vi "S4GUI_003.vi"(7 "Tab ObsEng":enum32{"Obs", "CCD modes", "Guider", "Eng"}(tab)) -> ()   [LabVIEW 2018] (continued)
            n4414 = call-dynamic "Read Channel.vi"("error in (no error)"=w10358, "Acquisition in"=w10359) -> ("error out"=w10342:errorcluster, "Channel.lvclass"=w10346:refnum<class "Channel.lvclass">, "Acquisition out"=w10352:refnum<class "Acquisition.lvclass">)  [unwired: 7 in]
            n4415 = call-dynamic "Read Interface.vi"("error in (no error)"=w10342, "Channel in"=w10346) -> ("error out"=w10337:errorcluster, "Interface.lvclass"=w10338:refnum<class "Interface.lvclass">, "Channel out"=w10345:refnum<class "Channel.lvclass">)  [unwired: 7 in]
            n4416 = call-dynamic "Write Cooler ON_OFF.vi"("error in (no error)"=w10337, "Cooler ON/OFF"=w10329, "Interface in"=w10338) -> ("error out"=w10341:errorcluster, "Interface out"=w10343:refnum<class "Interface.lvclass">)  [unwired: 7 in]
            n4417 = call-dynamic "Write Interface.vi"("error in (no error)"=w10341, "Interface.lvclass"=w10343, "Channel in"=w10345) -> ("error out"=w10340:errorcluster, "Channel out"=w10344:refnum<class "Channel.lvclass">)  [unwired: 7 in]
            n4418 = call-dynamic "Read State Machine.vi"("error in (no error)"=w10340, "Device in"=w10344) -> ("error out"=w10356:errorcluster, "State Machine.lvclass"=w10357:refnum<class "State Machine.lvclass">, "Device out"=w10353:refnum<class "Channel.lvclass">)  [unwired: 7 in]
            n4419 = call "Next State.vi"("error in (no error)"=w10356, "New_State"=u32 30, "State Machine in"=w10357) -> ("error out"=w10351:errorcluster, "State Machine out"=w10354:refnum<class "State Machine.lvclass">)  [unwired: 7 in]
            n4420 = call-dynamic "Write State Machine.vi"("error in (no error)"=w10351, "State Machine.lvclass"=w10354, "Device in"=w10353) -> ("error out"=w10347:errorcluster, "Device out"=w10339:refnum<class "Channel.lvclass">)  [unwired: 7 in]
            n4421 = call-dynamic "Write Channel.vi"("error in (no error)"=w10347, "Channel.lvclass"=w10339, "Acquisition in"=w10352) -> ("error out"=w10348:errorcluster, "Acquisition out"=w10350:refnum<class "Acquisition.lvclass">)  [unwired: 7 in]
            n4422 = call-dynamic "Write AcquisitionD.vi"("error in (no error)"=w10348, "Acquisition.lvclass"=w10350, "S4ACS_GUI in"=w10349) -> ("error out"=w10361:errorcluster, "S4ACS_GUI out"=w10360:refnum<class "S4GUI.lvclass">)  [unwired: 7 in]
          }
        }
      }
      event "Set Temp 1": Value Change {
        n4423 = event-data() -> ("NewVal"=w10362:bool)  [unwired: 1 in]
        n4424 = case shown="True" w10362 {
          tunnel: w10366 -> [w10368 w10385]
          tunnel: w10365 -> [w10367 w10384]
          tunnel: [w10367 w10374] -> w10364
          tunnel: [w10368 w10375] -> w10363
          frame False {
          }
          frame True {
            # "Carrega a maior temperatura\nentre target atual e o target do controle."
            # "Carrega o valor da temperatura target de acordo com a conf CCD"
            n4425 = call-dynamic "Read AcquisitionA.vi"("error in (no error)"=w10384, "S4ACS_GUI in"=w10385) -> ("error out"=w10387:errorcluster, "Acquisition.lvclass"=w10386:refnum<class "Acquisition.lvclass">, "S4ACS_GUI out"=w10371:refnum<class "S4GUI.lvclass">)  [unwired: 7 in]
            n4426 = call-dynamic "Read Channel.vi"("error in (no error)"=w10387, "Acquisition in"=w10386) -> ("error out"=w10398:errorcluster, "Channel.lvclass"=w10397:refnum<class "Channel.lvclass">, "Acquisition out"=w10370:refnum<class "Acquisition.lvclass">)  [unwired: 7 in]
            n4427 = call-dynamic "ValidateConfig.vi"("error in (no error)"=w10398, "Channel in"=w10397) -> ("error out"=w10404:errorcluster, "Channel out"=w10403:refnum<class "Channel.lvclass">)  [unwired: 7 in, 1 out]
            n4428 = call-dynamic "Read Interface.vi"("error in (no error)"=w10404, "Channel in"=w10403) -> ("error out"=w10400:errorcluster, "Interface.lvclass"=w10399:refnum<class "Interface.lvclass">, "Channel out"=w10393:refnum<class "Channel.lvclass">)  [unwired: 7 in]
            n4429 = call-dynamic "Read Temperature.vi"("error in (no error)"=w10400, "Interface in"=w10399) -> ("error out"=w10401:errorcluster, "Temperature"=w10405:i8, "Interface out"=w10402:refnum<class "Interface.lvclass">)  [unwired: 7 in]
            n4430 = Greater?(x=w10405, y="Target Temp 1") -> (0:w10373:bool)
            n4431 = Select(t=w10405, s=w10373, f="Target Temp 1") -> (s? t:f=w10378:i8)
            n4432 = call-dynamic "Write Temperature.vi"("error in (no error)"=w10401, "Temperature"=w10378, "Interface in"=w10402) -> ("error out"=w10395:errorcluster, "Interface out"=w10392:refnum<class "Interface.lvclass">)  [unwired: 7 in]
            n4433 = call-dynamic "Write Interface.vi"("error in (no error)"=w10395, "Interface.lvclass"=w10392, "Channel in"=w10393) -> ("error out"=w10396:errorcluster, "Channel out"=w10394:refnum<class "Channel.lvclass">)  [unwired: 7 in]
            n4434 = case shown="True" w10373 {
              tunnel: w10396 -> [w10430 w10433]
              tunnel: w10394 -> [w10429 w10440]
              tunnel: [w10428 w10440] -> w10391
              tunnel: [w10427 w10439] -> w10390
              tunnel: w10371 -> [w10407 w10435]
              tunnel: [w10407 w10438] -> w10372
              tunnel: w10370 -> [w10406 w10437]
              tunnel: [w10406 w10436] -> w10369
              frame False {
                # "input ok"
                n4435 = call-dynamic "Read State Machine.vi"("error in (no error)"=w10430, "Device in"=w10429) -> ("error out"=w10409:errorcluster, "State Machine.lvclass"=w10416:refnum<class "State Machine.lvclass">, "Device out"=w10425:refnum<class "Channel.lvclass">)  [unwired: 7 in]
                n4436 = call-dynamic "Read ref StatesQueue.vi"("error in (no error)"=w10409, "State Machine in"=w10416) -> ("error out"=w10419:errorcluster, "ref StatesQueue"=w10413:refnum<queue>, "State Machine out"=w10415:refnum<class "State Machine.lvclass">)  [unwired: 7 in]
                n4437 = Flush Queue(queue=w10413, error in (no error)=w10419) -> (queue out=w10412:refnum<queue>, error out=w10421:errorcluster)  [unwired: 1 out]
                n4438 = Enqueue Element(queue=w10412, element=u32 35 ("State"), error in (no error)=w10421) -> (queue out=w10411:refnum<queue>, error out=w10422:errorcluster)  [unwired: 1 in, 1 out]
                n4439 = Enqueue Element(queue=w10411, element=u32 37 ("State"), error in (no error)=w10422) -> (queue out=w10410:refnum<queue>, error out=w10420:errorcluster)  [unwired: 1 in, 1 out]
                n4440 = call-dynamic "Write ref StatesQueue.vi"("error in (no error)"=w10420, "ref StatesQueue"=w10410, "State Machine in"=w10415) -> ("error out"=w10408:errorcluster, "State Machine out"=w10414:refnum<class "State Machine.lvclass">)  [unwired: 7 in]
                n4441 = call "Next State.vi"("error in (no error)"=w10408, "New_State"=u32 0, "State Machine in"=w10414) -> ("error out"=w10426:errorcluster, "State Machine out"=w10424:refnum<class "State Machine.lvclass">)  [unwired: 7 in]
                n4442 = call-dynamic "Write State Machine.vi"("error in (no error)"=w10426, "State Machine.lvclass"=w10424, "Device in"=w10425) -> ("error out"=w10427:errorcluster, "Device out"=w10428:refnum<class "Channel.lvclass">)  [unwired: 7 in]
              }
              frame True {
                # "input error"
                n4443 = call-dynamic "Read SET temp error mode.vi"("error in (no error)"=w10433, "S4GUI in"=w10435) -> ("error out"=w10432:errorcluster, "SET temp error mode"=w10431:bool, "S4GUI out"=w10434:refnum<class "S4GUI.lvclass">)  [unwired: 7 in]
                n4444 = case shown="False" w10431 {
                  tunnel: [w10449 w10464] -> w10439
                  tunnel: [w10448 w10463] -> w10438
                  tunnel: w10434 -> [w10447 w10463]
                  tunnel: w10432 -> [w10444 w10465]
                  tunnel: w10437 -> [w10442 w10462]
                  tunnel: [w10441 w10462] -> w10436
                  frame False {
                    # "last error msg"
                    n4445 = call-dynamic "Read sync.vi"("error in (no error)"=w10444, "S4ACS_GUI in"=w10447) -> ("error out"=w10443:errorcluster, "sync"=w10445:bool, "S4ACS_GUI out"=w10446:refnum<class "S4GUI.lvclass">)  [unwired: 7 in]
                    n4446 = case shown="False" w10445 {
                      tunnel: w10443 -> [w10452 w10461]
                      tunnel: [w10451 w10460] -> w10449
                      tunnel: [w10455 w10459] -> w10448
                      tunnel: w10446 -> [w10455 w10457]
                      tunnel: w10442 -> [w10453 w10456]
                      tunnel: [w10450 w10456] -> w10441
                      frame False {
                        n4447 = call-dynamic "Write Acq_state.vi"("error in (no error)"=w10452, "Acq_state"=u32 240, "Acquisition in"=w10453) -> ("error out"=w10451:errorcluster, "Acquisition out"=w10450:refnum<class "Acquisition.lvclass">)  [unwired: 7 in]
                      }
                      frame True {
                        n4448 = call-dynamic "Write Obs_state.vi"("error in (no error)"=w10461, "Obs_state"=u32 240, "S4ACS_GUI in"=w10457) -> ("error out"=w10460:errorcluster, "S4ACS_GUI out"=w10459:refnum<class "S4GUI.lvclass">)  [unwired: 7 in]
                      }
                    }
                  }
                  frame True {
                    # "popup msg"
                    n4449 = disable-structure shown="Enabled" {
                      disable-tunnel: w10465 -> [w10467 w10474]
                      disable-tunnel: [w10466 w10474] -> w10464
                      frame Enabled {
                        w10469 = FALSE ("Wait Until Done")
                        n4450 = call <vilib>:"Application Directory.vi"() -> ("Application Directory"=w10473:path)
                        n4451 = Build Path(base path=w10473, name or relative path="MsgSetTemp.vi") -> (appended path=w10470:path)
                        n4452 = Open VI Reference(vi path=w10470, error in (no error)=w10467) -> (vi reference=w10471:refnum<vi>, error out=w10472:errorcluster)  [unwired: 4 in]
                        n4453 = invoke class="VI" method="Run VI"(reference=w10471, error in=w10472, "Wait until done"=w10469, "Auto Dispose Ref"=w10469) -> (error out=w10466:errorcluster)  [unwired: 1 in, 4 out]
                      }
                      frame Disabled {
                        n4454 = One Button Dialog(message="ERROR: Invalid input value. It must be \nequal or greater than the minimum for \nthe current CCD setup.", button name ("OK")="OK" ("T button name (\"OK\")")) -> ()  [unwired: 1 out]
                      }
                    }
                  }
                }
              }
            }
            n4455 = Number To Decimal String(number="Target Temp 1") -> (decimal integer string=w10377:string)  [unwired: 1 in]
            n4456 = call-dynamic "Write Channel.vi"("error in (no error)"=w10390, "Channel.lvclass"=w10391, "Acquisition in"=w10369) -> ("error out"=w10389:errorcluster, "Acquisition out"=w10388:refnum<class "Acquisition.lvclass">)  [unwired: 7 in]
            n4457 = Concatenate Strings("SET TEMP [" ("User Event"), w10377, "] CLICKED - CH1" ("User Event")) -> (w10383:string)
            n4458 = call-dynamic "Write AcquisitionA.vi"("error in (no error)"=w10389, "Acquisition.lvclass"=w10388, "S4ACS_GUI in"=w10372) -> ("error out"=w10379:errorcluster, "S4ACS_GUI out"=w10380:refnum<class "S4GUI.lvclass">)  [unwired: 7 in]
            n4459 = call-dynamic "Write User Event.vi"("error in (no error)"=w10379, "User Event"=w10383, "S4GUI in"=w10380) -> ("error out"=w10374:errorcluster, "S4GUI out"=w10375:refnum<class "S4GUI.lvclass">)  [unwired: 7 in]
          }
        }
      }
      event "Set Temp 2": Value Change {
        n4460 = event-data() -> ("NewVal"=w10477:bool)  [unwired: 1 in]
        n4461 = case shown="True" w10477 {
          tunnel: w10481 -> [w10483 w10503]
          tunnel: w10480 -> [w10482 w10502]
          tunnel: [w10482 w10495] -> w10479
          tunnel: [w10483 w10497] -> w10478
          frame False {
          }
          frame True {
            # "Carrega a maior temperatura\nentre target atual e o target do controle."
            # "Carrega o valor da temperatura target de acordo com a conf CCD"
            n4462 = call "Read AcquisitionB.vi"("error in (no error)"=w10502, "S4ACS_GUI in"=w10503) -> ("error out"=w10519:errorcluster, "Acquisition.lvclass"=w10520:refnum<class "Acquisition.lvclass">, "S4ACS_GUI out"=w10490:refnum<class "S4GUI.lvclass">)  [unwired: 7 in]
            n4463 = call-dynamic "Read Channel.vi"("error in (no error)"=w10519, "Acquisition in"=w10520) -> ("error out"=w10512:errorcluster, "Channel.lvclass"=w10513:refnum<class "Channel.lvclass">, "Acquisition out"=w10491:refnum<class "Acquisition.lvclass">)  [unwired: 7 in]
            n4464 = call-dynamic "ValidateConfig.vi"("error in (no error)"=w10512, "Channel in"=w10513) -> ("error out"=w10506:errorcluster, "Channel out"=w10507:refnum<class "Channel.lvclass">)  [unwired: 7 in, 1 out]
            n4465 = call-dynamic "Read Interface.vi"("error in (no error)"=w10506, "Channel in"=w10507) -> ("error out"=w10510:errorcluster, "Interface.lvclass"=w10511:refnum<class "Interface.lvclass">, "Channel out"=w10515:refnum<class "Channel.lvclass">)  [unwired: 7 in]
            n4466 = call-dynamic "Read Temperature.vi"("error in (no error)"=w10510, "Interface in"=w10511) -> ("error out"=w10509:errorcluster, "Temperature"=w10505:i8, "Interface out"=w10508:refnum<class "Interface.lvclass">)  [unwired: 7 in]
            n4467 = Greater?(x=w10505, y="Target Temp 2") -> (0:w10488:bool)
            n4468 = Select(t=w10505, s=w10488, f="Target Temp 2") -> (s? t:f=w10504:i32)
            n4469 = call-dynamic "Write Temperature.vi"("error in (no error)"=w10509, "Temperature"=w10504, "Interface in"=w10508) -> ("error out"=w10514:errorcluster, "Interface out"=w10516:refnum<class "Interface.lvclass">)  [unwired: 7 in]
            n4470 = call-dynamic "Write Interface.vi"("error in (no error)"=w10514, "Interface.lvclass"=w10516, "Channel in"=w10515) -> ("error out"=w10489:errorcluster, "Channel out"=w10492:refnum<class "Channel.lvclass">)  [unwired: 7 in]
            n4471 = case shown="True" w10488 {
              tunnel: w10489 -> [w10545 w10550]
              tunnel: w10492 -> [w10544 w10552]
              tunnel: [w10543 w10552] -> w10485
              tunnel: [w10542 w10555] -> w10484
              tunnel: w10490 -> [w10522 w10551]
              tunnel: [w10522 w10554] -> w10487
              tunnel: w10491 -> [w10521 w10546]
              tunnel: [w10521 w10553] -> w10486
              frame False {
                # "input ok"
                n4472 = call-dynamic "Read State Machine.vi"("error in (no error)"=w10545, "Device in"=w10544) -> ("error out"=w10524:errorcluster, "State Machine.lvclass"=w10531:refnum<class "State Machine.lvclass">, "Device out"=w10540:refnum<class "Channel.lvclass">)  [unwired: 7 in]
                n4473 = call-dynamic "Read ref StatesQueue.vi"("error in (no error)"=w10524, "State Machine in"=w10531) -> ("error out"=w10534:errorcluster, "ref StatesQueue"=w10528:refnum<queue>, "State Machine out"=w10530:refnum<class "State Machine.lvclass">)  [unwired: 7 in]
                n4474 = Flush Queue(queue=w10528, error in (no error)=w10534) -> (queue out=w10527:refnum<queue>, error out=w10536:errorcluster)  [unwired: 1 out]
                n4475 = Enqueue Element(queue=w10527, element=u32 35 ("State"), error in (no error)=w10536) -> (queue out=w10526:refnum<queue>, error out=w10537:errorcluster)  [unwired: 1 in, 1 out]
                n4476 = Enqueue Element(queue=w10526, element=u32 37 ("State"), error in (no error)=w10537) -> (queue out=w10525:refnum<queue>, error out=w10535:errorcluster)  [unwired: 1 in, 1 out]
                n4477 = call-dynamic "Write ref StatesQueue.vi"("error in (no error)"=w10535, "ref StatesQueue"=w10525, "State Machine in"=w10530) -> ("error out"=w10523:errorcluster, "State Machine out"=w10529:refnum<class "State Machine.lvclass">)  [unwired: 7 in]
                n4478 = call "Next State.vi"("error in (no error)"=w10523, "New_State"=u32 0, "State Machine in"=w10529) -> ("error out"=w10541:errorcluster, "State Machine out"=w10539:refnum<class "State Machine.lvclass">)  [unwired: 7 in]
                n4479 = call-dynamic "Write State Machine.vi"("error in (no error)"=w10541, "State Machine.lvclass"=w10539, "Device in"=w10540) -> ("error out"=w10542:errorcluster, "Device out"=w10543:refnum<class "Channel.lvclass">)  [unwired: 7 in]
              }
              frame True {
                # "input error"
                n4480 = call-dynamic "Read SET temp error mode.vi"("error in (no error)"=w10550, "S4GUI in"=w10551) -> ("error out"=w10547:errorcluster, "SET temp error mode"=w10549:bool, "S4GUI out"=w10548:refnum<class "S4GUI.lvclass">)  [unwired: 7 in]
                n4481 = case shown="False" w10549 {
                  tunnel: [w10564 w10577] -> w10555
                  tunnel: [w10563 w10586] -> w10554
                  tunnel: [w10559 w10585] -> w10553
                  tunnel: w10546 -> [w10558 w10585]
                  tunnel: w10548 -> [w10557 w10586]
                  tunnel: w10547 -> [w10556 w10578]
                  frame False {
                    # "last error msg"
                    n4482 = call-dynamic "Read sync.vi"("error in (no error)"=w10556, "S4ACS_GUI in"=w10557) -> ("error out"=w10560:errorcluster, "sync"=w10561:bool, "S4ACS_GUI out"=w10562:refnum<class "S4GUI.lvclass">)  [unwired: 7 in]
                    n4483 = case shown="True" w10561 {
                      tunnel: w10560 -> [w10567 w10576]
                      tunnel: [w10566 w10575] -> w10564
                      tunnel: [w10570 w10574] -> w10563
                      tunnel: w10562 -> [w10570 w10572]
                      tunnel: w10558 -> [w10568 w10571]
                      tunnel: [w10565 w10571] -> w10559
                      frame False {
                        n4484 = call-dynamic "Write Acq_state.vi"("error in (no error)"=w10567, "Acq_state"=u32 240, "Acquisition in"=w10568) -> ("error out"=w10566:errorcluster, "Acquisition out"=w10565:refnum<class "Acquisition.lvclass">)  [unwired: 7 in]
                      }
                      frame True {
                        n4485 = call-dynamic "Write Obs_state.vi"("error in (no error)"=w10576, "Obs_state"=u32 240, "S4ACS_GUI in"=w10572) -> ("error out"=w10575:errorcluster, "S4ACS_GUI out"=w10574:refnum<class "S4GUI.lvclass">)  [unwired: 7 in]
                      }
                    }
                  }
                  frame True {
                    w10580 = FALSE ("Wait Until Done")
                    # "popup msg"
                    n4486 = call <vilib>:"Application Directory.vi"() -> ("Application Directory"=w10584:path)
                    n4487 = Build Path(base path=w10584, name or relative path="MsgSetTemp.vi") -> (appended path=w10581:path)
                    n4488 = Open VI Reference(vi path=w10581, error in (no error)=w10578) -> (vi reference=w10582:refnum<vi>, error out=w10583:errorcluster)  [unwired: 4 in]
                    n4489 = invoke class="VI" method="Run VI"(reference=w10582, error in=w10583, "Wait until done"=w10580, "Auto Dispose Ref"=w10580) -> (error out=w10577:errorcluster)  [unwired: 1 in, 4 out]
                  }
                }
              }
            }
            n4490 = Number To Decimal String(number="Target Temp 2") -> (decimal integer string=w10493:string)  [unwired: 1 in]
            n4491 = call-dynamic "Write Channel.vi"("error in (no error)"=w10484, "Channel.lvclass"=w10485, "Acquisition in"=w10486) -> ("error out"=w10517:errorcluster, "Acquisition out"=w10518:refnum<class "Acquisition.lvclass">)  [unwired: 7 in]
            n4492 = Concatenate Strings("SET TEMP [" ("User Event"), w10493, "] CLICKED - CH2" ("User Event")) -> (w10501:string)
            n4493 = call "Write AcquisitionB.vi"("error in (no error)"=w10517, "Acquisition.lvclass"=w10518, "S4ACS_GUI in"=w10487) -> ("error out"=w10496:errorcluster, "S4ACS_GUI out"=w10498:refnum<class "S4GUI.lvclass">)  [unwired: 7 in]
            n4494 = call-dynamic "Write User Event.vi"("error in (no error)"=w10496, "User Event"=w10501, "S4GUI in"=w10498) -> ("error out"=w10495:errorcluster, "S4GUI out"=w10497:refnum<class "S4GUI.lvclass">)  [unwired: 7 in]
          }
        }
      }
      event "Set Temp 3": Value Change {
        n4495 = event-data() -> ("NewVal"=w10587:bool)  [unwired: 1 in]
        n4496 = case shown="True" w10587 {
          tunnel: w10591 -> [w10593 w10613]
          tunnel: w10590 -> [w10592 w10612]
          tunnel: [w10592 w10604] -> w10589
          tunnel: [w10593 w10606] -> w10588
          frame False {
          }
          frame True {
            # "Carrega a maior temperatura\nentre target atual e o target do controle."
            # "Carrega o valor da temperatura target de acordo com a conf CCD"
            n4497 = call-dynamic "Read AcquisitionC.vi"("error in (no error)"=w10612, "S4ACS_GUI in"=w10613) -> ("error out"=w10615:errorcluster, "Acquisition.lvclass"=w10614:refnum<class "Acquisition.lvclass">, "S4ACS_GUI out"=w10595:refnum<class "S4GUI.lvclass">)  [unwired: 7 in]
            n4498 = call-dynamic "Read Channel.vi"("error in (no error)"=w10615, "Acquisition in"=w10614) -> ("error out"=w10622:errorcluster, "Channel.lvclass"=w10621:refnum<class "Channel.lvclass">, "Acquisition out"=w10596:refnum<class "Acquisition.lvclass">)  [unwired: 7 in]
            n4499 = call-dynamic "ValidateConfig.vi"("error in (no error)"=w10622, "Channel in"=w10621) -> ("error out"=w10628:errorcluster, "Channel out"=w10627:refnum<class "Channel.lvclass">)  [unwired: 7 in, 1 out]
            n4500 = call-dynamic "Read Interface.vi"("error in (no error)"=w10628, "Channel in"=w10627) -> ("error out"=w10624:errorcluster, "Interface.lvclass"=w10623:refnum<class "Interface.lvclass">, "Channel out"=w10619:refnum<class "Channel.lvclass">)  [unwired: 7 in]
            n4501 = call-dynamic "Read Temperature.vi"("error in (no error)"=w10624, "Interface in"=w10623) -> ("error out"=w10625:errorcluster, "Temperature"=w10629:i8, "Interface out"=w10626:refnum<class "Interface.lvclass">)  [unwired: 7 in]
            n4502 = Greater?(x=w10629, y="Target Temp 3") -> (0:w10594:bool)
            n4503 = Select(t=w10629, s=w10594, f="Target Temp 3") -> (s? t:f=w10630:i32)
            n4504 = call-dynamic "Write Temperature.vi"("error in (no error)"=w10625, "Temperature"=w10630, "Interface in"=w10626) -> ("error out"=w10620:errorcluster, "Interface out"=w10618:refnum<class "Interface.lvclass">)  [unwired: 7 in]
            n4505 = call-dynamic "Write Interface.vi"("error in (no error)"=w10620, "Interface.lvclass"=w10618, "Channel in"=w10619) -> ("error out"=w10597:errorcluster, "Channel out"=w10602:refnum<class "Channel.lvclass">)  [unwired: 7 in]
            n4506 = case shown="True" w10594 {
              tunnel: w10597 -> [w10655 w10656]
              tunnel: w10602 -> [w10654 w10662]
              tunnel: [w10653 w10662] -> w10601
              tunnel: [w10652 w10665] -> w10598
              tunnel: w10595 -> [w10632 w10661]
              tunnel: [w10632 w10664] -> w10599
              tunnel: w10596 -> [w10631 w10659]
              tunnel: [w10631 w10663] -> w10600
              frame False {
                # "input ok"
                n4507 = call-dynamic "Read State Machine.vi"("error in (no error)"=w10655, "Device in"=w10654) -> ("error out"=w10634:errorcluster, "State Machine.lvclass"=w10641:refnum<class "State Machine.lvclass">, "Device out"=w10650:refnum<class "Channel.lvclass">)  [unwired: 7 in]
                n4508 = call-dynamic "Read ref StatesQueue.vi"("error in (no error)"=w10634, "State Machine in"=w10641) -> ("error out"=w10644:errorcluster, "ref StatesQueue"=w10638:refnum<queue>, "State Machine out"=w10640:refnum<class "State Machine.lvclass">)  [unwired: 7 in]
                n4509 = Flush Queue(queue=w10638, error in (no error)=w10644) -> (queue out=w10637:refnum<queue>, error out=w10646:errorcluster)  [unwired: 1 out]
                n4510 = Enqueue Element(queue=w10637, element=u32 35 ("State"), error in (no error)=w10646) -> (queue out=w10636:refnum<queue>, error out=w10647:errorcluster)  [unwired: 1 in, 1 out]
                n4511 = Enqueue Element(queue=w10636, element=u32 37 ("State"), error in (no error)=w10647) -> (queue out=w10635:refnum<queue>, error out=w10645:errorcluster)  [unwired: 1 in, 1 out]
                n4512 = call-dynamic "Write ref StatesQueue.vi"("error in (no error)"=w10645, "ref StatesQueue"=w10635, "State Machine in"=w10640) -> ("error out"=w10633:errorcluster, "State Machine out"=w10639:refnum<class "State Machine.lvclass">)  [unwired: 7 in]
                n4513 = call "Next State.vi"("error in (no error)"=w10633, "New_State"=u32 0, "State Machine in"=w10639) -> ("error out"=w10651:errorcluster, "State Machine out"=w10649:refnum<class "State Machine.lvclass">)  [unwired: 7 in]
                n4514 = call-dynamic "Write State Machine.vi"("error in (no error)"=w10651, "State Machine.lvclass"=w10649, "Device in"=w10650) -> ("error out"=w10652:errorcluster, "Device out"=w10653:refnum<class "Channel.lvclass">)  [unwired: 7 in]
              }
              frame True {
                # "input error"
                n4515 = call-dynamic "Read SET temp error mode.vi"("error in (no error)"=w10656, "S4GUI in"=w10661) -> ("error out"=w10657:errorcluster, "SET temp error mode"=w10658:bool, "S4GUI out"=w10660:refnum<class "S4GUI.lvclass">)  [unwired: 7 in]
                n4516 = case shown="False" w10658 {
                  tunnel: [w10674 w10687] -> w10665
                  tunnel: [w10673 w10696] -> w10664
                  tunnel: w10660 -> [w10672 w10696]
                  tunnel: w10657 -> [w10669 w10688]
                  tunnel: w10659 -> [w10667 w10695]
                  tunnel: [w10666 w10695] -> w10663
                  frame False {
                    # "last error msg"
                    n4517 = call-dynamic "Read sync.vi"("error in (no error)"=w10669, "S4ACS_GUI in"=w10672) -> ("error out"=w10668:errorcluster, "sync"=w10670:bool, "S4ACS_GUI out"=w10671:refnum<class "S4GUI.lvclass">)  [unwired: 7 in]
                    n4518 = case shown="True" w10670 {
                      tunnel: w10668 -> [w10677 w10686]
                      tunnel: [w10676 w10685] -> w10674
                      tunnel: [w10680 w10684] -> w10673
                      tunnel: w10671 -> [w10680 w10682]
                      tunnel: w10667 -> [w10678 w10681]
                      tunnel: [w10675 w10681] -> w10666
                      frame False {
                        n4519 = call-dynamic "Write Acq_state.vi"("error in (no error)"=w10677, "Acq_state"=u32 240, "Acquisition in"=w10678) -> ("error out"=w10676:errorcluster, "Acquisition out"=w10675:refnum<class "Acquisition.lvclass">)  [unwired: 7 in]
                      }
                      frame True {
                        n4520 = call-dynamic "Write Obs_state.vi"("error in (no error)"=w10686, "Obs_state"=u32 240, "S4ACS_GUI in"=w10682) -> ("error out"=w10685:errorcluster, "S4ACS_GUI out"=w10684:refnum<class "S4GUI.lvclass">)  [unwired: 7 in]
                      }
                    }
                  }
                  frame True {
                    w10690 = FALSE ("Wait Until Done")
                    # "popup msg"
                    n4521 = call <vilib>:"Application Directory.vi"() -> ("Application Directory"=w10691:path)
                    n4522 = Build Path(base path=w10691, name or relative path="MsgSetTemp.vi") -> (appended path=w10694:path)
                    n4523 = Open VI Reference(vi path=w10694, error in (no error)=w10688) -> (vi reference=w10693:refnum<vi>, error out=w10692:errorcluster)  [unwired: 4 in]
                    n4524 = invoke class="VI" method="Run VI"(reference=w10693, error in=w10692, "Wait until done"=w10690, "Auto Dispose Ref"=w10690) -> (error out=w10687:errorcluster)  [unwired: 1 in, 4 out]
                  }
                }
              }
            }
            n4525 = Number To Decimal String(number="Target Temp 3") -> (decimal integer string=w10608:string)  [unwired: 1 in]
            n4526 = call-dynamic "Write Channel.vi"("error in (no error)"=w10598, "Channel.lvclass"=w10601, "Acquisition in"=w10600) -> ("error out"=w10617:errorcluster, "Acquisition out"=w10616:refnum<class "Acquisition.lvclass">)  [unwired: 7 in]
            n4527 = call-dynamic "Write AcquisitionC.vi"("error in (no error)"=w10617, "Acquisition.lvclass"=w10616, "S4ACS_GUI in"=w10599) -> ("error out"=w10605:errorcluster, "S4ACS_GUI out"=w10607:refnum<class "S4GUI.lvclass">)  [unwired: 7 in]
            n4528 = Concatenate Strings("SET TEMP [" ("User Event"), w10608, "] CLICKED - CH3" ("User Event")) -> (w10611:string)
            n4529 = call-dynamic "Write User Event.vi"("error in (no error)"=w10605, "User Event"=w10611, "S4GUI in"=w10607) -> ("error out"=w10604:errorcluster, "S4GUI out"=w10606:refnum<class "S4GUI.lvclass">)  [unwired: 7 in]
          }
        }
      }
      event "Set Temp 4": Value Change {
        n4530 = event-data() -> ("NewVal"=w10697:bool)  [unwired: 1 in]
        n4531 = case shown="True" w10697 {
          tunnel: w10701 -> [w10703 w10736]
          tunnel: w10700 -> [w10702 w10735]
          tunnel: [w10702 w10713] -> w10699
          tunnel: [w10703 w10714] -> w10698
          frame False {
          }
          frame True {
            # "Carrega a maior temperatura\nentre target atual e o target do controle."
            # "Carrega o valor da temperatura target de acordo com a conf CCD"
            n4532 = call-dynamic "Read AcquisitionD.vi"("error in (no error)"=w10735, "S4ACS_GUI in"=w10736) -> ("error out"=w10739:errorcluster, "Acquisition.lvclass"=w10740:refnum<class "Acquisition.lvclass">, "S4ACS_GUI out"=w10709:refnum<class "S4GUI.lvclass">)  [unwired: 7 in]
            n4533 = call-dynamic "Read Channel.vi"("error in (no error)"=w10739, "Acquisition in"=w10740) -> ("error out"=w10730:errorcluster, "Channel.lvclass"=w10731:refnum<class "Channel.lvclass">, "Acquisition out"=w10710:refnum<class "Acquisition.lvclass">)  [unwired: 7 in]
            n4534 = call-dynamic "ValidateConfig.vi"("error in (no error)"=w10730, "Channel in"=w10731) -> ("error out"=w10724:errorcluster, "Channel out"=w10725:refnum<class "Channel.lvclass">)  [unwired: 7 in, 1 out]
            n4535 = call-dynamic "Read Interface.vi"("error in (no error)"=w10724, "Channel in"=w10725) -> ("error out"=w10728:errorcluster, "Interface.lvclass"=w10729:refnum<class "Interface.lvclass">, "Channel out"=w10733:refnum<class "Channel.lvclass">)  [unwired: 7 in]
            n4536 = call-dynamic "Read Temperature.vi"("error in (no error)"=w10728, "Interface in"=w10729) -> ("error out"=w10727:errorcluster, "Temperature"=w10723:i8, "Interface out"=w10726:refnum<class "Interface.lvclass">)  [unwired: 7 in]
            n4537 = Greater?(x=w10723, y="Target Temp 4") -> (0:w10708:bool)
            n4538 = Select(t=w10723, s=w10708, f="Target Temp 4") -> (s? t:f=w10722:i32)
            n4539 = call-dynamic "Write Temperature.vi"("error in (no error)"=w10727, "Temperature"=w10722, "Interface in"=w10726) -> ("error out"=w10732:errorcluster, "Interface out"=w10734:refnum<class "Interface.lvclass">)  [unwired: 7 in]
            n4540 = call-dynamic "Write Interface.vi"("error in (no error)"=w10732, "Interface.lvclass"=w10734, "Channel in"=w10733) -> ("error out"=w10711:errorcluster, "Channel out"=w10712:refnum<class "Channel.lvclass">)  [unwired: 7 in]
            n4541 = case shown="True" w10708 {
              tunnel: w10711 -> [w10765 w10770]
              tunnel: w10712 -> [w10764 w10772]
              tunnel: [w10763 w10772] -> w10707
              tunnel: [w10762 w10775] -> w10704
              tunnel: w10709 -> [w10742 w10771]
              tunnel: [w10742 w10774] -> w10705
              tunnel: w10710 -> [w10741 w10767]
              tunnel: [w10741 w10773] -> w10706
              frame False {
                n4542 = call-dynamic "Read State Machine.vi"("error in (no error)"=w10765, "Device in"=w10764) -> ("error out"=w10744:errorcluster, "State Machine.lvclass"=w10751:refnum<class "State Machine.lvclass">, "Device out"=w10760:refnum<class "Channel.lvclass">)  [unwired: 7 in]
                n4543 = call-dynamic "Read ref StatesQueue.vi"("error in (no error)"=w10744, "State Machine in"=w10751) -> ("error out"=w10754:errorcluster, "ref StatesQueue"=w10748:refnum<queue>, "State Machine out"=w10750:refnum<class "State Machine.lvclass">)  [unwired: 7 in]
                n4544 = Flush Queue(queue=w10748, error in (no error)=w10754) -> (queue out=w10747:refnum<queue>, error out=w10756:errorcluster)  [unwired: 1 out]
                n4545 = Enqueue Element(queue=w10747, element=u32 35 ("State"), error in (no error)=w10756) -> (queue out=w10746:refnum<queue>, error out=w10757:errorcluster)  [unwired: 1 in, 1 out]
                n4546 = Enqueue Element(queue=w10746, element=u32 37 ("State"), error in (no error)=w10757) -> (queue out=w10745:refnum<queue>, error out=w10755:errorcluster)  [unwired: 1 in, 1 out]
                n4547 = call-dynamic "Write ref StatesQueue.vi"("error in (no error)"=w10755, "ref StatesQueue"=w10745, "State Machine in"=w10750) -> ("error out"=w10743:errorcluster, "State Machine out"=w10749:refnum<class "State Machine.lvclass">)  [unwired: 7 in]
                n4548 = call "Next State.vi"("error in (no error)"=w10743, "New_State"=u32 0, "State Machine in"=w10749) -> ("error out"=w10761:errorcluster, "State Machine out"=w10759:refnum<class "State Machine.lvclass">)  [unwired: 7 in]
                n4549 = call-dynamic "Write State Machine.vi"("error in (no error)"=w10761, "State Machine.lvclass"=w10759, "Device in"=w10760) -> ("error out"=w10762:errorcluster, "Device out"=w10763:refnum<class "Channel.lvclass">)  [unwired: 7 in]
              }
              frame True {
                # "input error"
                n4550 = call-dynamic "Read SET temp error mode.vi"("error in (no error)"=w10770, "S4GUI in"=w10771) -> ("error out"=w10769:errorcluster, "SET temp error mode"=w10766:bool, "S4GUI out"=w10768:refnum<class "S4GUI.lvclass">)  [unwired: 7 in]
                n4551 = case shown="True" w10766 {
                  tunnel: [w10784 w10797] -> w10775
                  tunnel: [w10783 w10805] -> w10774
                  tunnel: [w10779 w10804] -> w10773
                  tunnel: w10769 -> [w10778 w10797]
                  tunnel: w10768 -> [w10776 w10805]
                  tunnel: w10767 -> [w10777 w10804]
                  frame False {
                    # "last error msg"
                    n4552 = call-dynamic "Read sync.vi"("error in (no error)"=w10778, "S4ACS_GUI in"=w10776) -> ("error out"=w10780:errorcluster, "sync"=w10781:bool, "S4ACS_GUI out"=w10782:refnum<class "S4GUI.lvclass">)  [unwired: 7 in]
                    n4553 = case shown="False" w10781 {
                      tunnel: w10780 -> [w10787 w10796]
                      tunnel: [w10786 w10795] -> w10784
                      tunnel: [w10790 w10794] -> w10783
                      tunnel: w10782 -> [w10790 w10792]
                      tunnel: w10777 -> [w10788 w10791]
                      tunnel: [w10785 w10791] -> w10779
                      frame False {
                        n4554 = call-dynamic "Write Acq_state.vi"("error in (no error)"=w10787, "Acq_state"=u32 240, "Acquisition in"=w10788) -> ("error out"=w10786:errorcluster, "Acquisition out"=w10785:refnum<class "Acquisition.lvclass">)  [unwired: 7 in]
                      }
                      frame True {
                        n4555 = call-dynamic "Write Obs_state.vi"("error in (no error)"=w10796, "Obs_state"=u32 240, "S4ACS_GUI in"=w10792) -> ("error out"=w10795:errorcluster, "S4ACS_GUI out"=w10794:refnum<class "S4GUI.lvclass">)  [unwired: 7 in]
                      }
                    }
                  }
                  frame True {
                    w10799 = FALSE ("Wait Until Done")
                    # "popup msg"
                    n4556 = call <vilib>:"Application Directory.vi"() -> ("Application Directory"=w10803:path)
                    n4557 = Build Path(base path=w10803, name or relative path="MsgSetTemp.vi") -> (appended path=w10800:path)
                    n4558 = Open VI Reference(vi path=w10800) -> (vi reference=w10801:refnum<vi>, error out=w10802:errorcluster)  [unwired: 5 in]
                    n4559 = invoke class="VI" method="Run VI"(reference=w10801, error in=w10802, "Wait until done"=w10799, "Auto Dispose Ref"=w10799) -> ()  [unwired: 1 in, 5 out]
                  }
                }
              }
            }
            n4560 = Number To Decimal String(number="Target Temp 4") -> (decimal integer string=w10721:string)  [unwired: 1 in]
            n4561 = call-dynamic "Write Channel.vi"("error in (no error)"=w10704, "Channel.lvclass"=w10707, "Acquisition in"=w10706) -> ("error out"=w10737:errorcluster, "Acquisition out"=w10738:refnum<class "Acquisition.lvclass">)  [unwired: 7 in]
            n4562 = Concatenate Strings("SET TEMP [" ("User Event"), w10721, "] CLICKED - CH4" ("User Event")) -> (w10720:string)
            n4563 = call-dynamic "Write AcquisitionD.vi"("error in (no error)"=w10737, "Acquisition.lvclass"=w10738, "S4ACS_GUI in"=w10705) -> ("error out"=w10715:errorcluster, "S4ACS_GUI out"=w10716:refnum<class "S4GUI.lvclass">)  [unwired: 7 in]
            n4564 = call-dynamic "Write User Event.vi"("error in (no error)"=w10715, "User Event"=w10720, "S4GUI in"=w10716) -> ("error out"=w10713:errorcluster, "S4GUI out"=w10714:refnum<class "S4GUI.lvclass">)  [unwired: 7 in]
          }
        }
      }
      event "SET Temp message": Value Change {
        # "Seleção do modo de apresentação da\nmensagem de erro para o SET de \ntemperatura manual:\nF: via Last Error em vermelho (S4GUI:HandleObservation.vi);\nT: via janela de popup (MsgTempPopup.vi)."
        n4565 = event-data() -> ("NewVal"=w10808:bool)  [unwired: 1 in]
        n4566 = call-dynamic "Write SET temp error mode.vi"("error in (no error)"=w10809, "SET temp error mode"=w10808, "S4GUI in"=w10810) -> ("error out"=w10806:errorcluster, "S4GUI out"=w10807:refnum<class "S4GUI.lvclass">)  [unwired: 7 in]
      }
      event "Avança Estado": Value Change {
        n4567 = event-data() -> ()  [unwired: 1 in, 4 out]
        n4568 = call-dynamic "Read Sync Box.lvclass.vi"("error in (no error)"=w10819, "SPARC4_AC in"=w10820) -> ("error out"=w10832:errorcluster, "Sync Box.lvclass"=w10833:refnum<class "Sync Box.lvclass">, "SPARC4_AC out"=w10824:refnum<class "S4GUI.lvclass">)  [unwired: 7 in]
        n4569 = call-dynamic "Read Trigger.lvclass.vi"("error in (no error)"=w10832, "Sync Box in"=w10833) -> ("error out"=w10830:errorcluster, "Trigger.lvclass"=w10831:refnum<class "Trigger.lvclass">, "Sync Box out"=w10827:refnum<class "Sync Box.lvclass">)  [unwired: 7 in]
        n4570 = call-dynamic "Read State Machine.vi"("error in (no error)"=w10830, "Device in"=w10831) -> ("error out"=w10816:errorcluster, "State Machine.lvclass"=w10817:refnum<class "State Machine.lvclass">, "Device out"=w10828:refnum<class "Trigger.lvclass">)  [unwired: 7 in]
        n4571 = call-dynamic "Read State.vi"("error in (no error)"=w10816, "State Machine in"=w10817) -> ("error out"=w10812:errorcluster, "State"=w10815:i32, "State Machine out"=w10813:refnum<class "State Machine.lvclass">)  [unwired: 7 in]
        n4572 = Increment(x=w10815) -> (x+1=w10814:i32)
        n4573 = call "Next State.vi"("error in (no error)"=w10812, "New_State"=w10814, "State Machine in"=w10813) -> ("error out"=w10826:errorcluster, "State Machine out"=w10829:refnum<class "State Machine.lvclass">)  [unwired: 7 in]
        n4574 = call-dynamic "Write State Machine.vi"("error in (no error)"=w10826, "State Machine.lvclass"=w10829, "Device in"=w10828) -> ("error out"=w10822:errorcluster, "Device out"=w10821:refnum<class "Trigger.lvclass">)  [unwired: 7 in]
        n4575 = call-dynamic "Write Trigger.lvclass.vi"("error in (no error)"=w10822, "Trigger.lvclass"=w10821, "Sync Box in"=w10827) -> ("error out"=w10823:errorcluster, "Sync Box out"=w10825:refnum<class "Sync Box.lvclass">)  [unwired: 7 in]
        n4576 = call-dynamic "Write Sync Box.lvclass.vi"("error in (no error)"=w10823, "Sync Box.lvclass"=w10825, "SPARC4_AC in"=w10824) -> ("error out"=w10818:errorcluster, "SPARC4_AC out"=w10811:refnum<class "S4GUI.lvclass">)  [unwired: 7 in]
      }
      event "DelayA": Value Change {
        n4577 = event-data() -> ("NewVal"=w10835:string)  [unwired: 1 in, 3 out]
        n4578 = call-dynamic "Read Sync Box.lvclass.vi"("error in (no error)"=w10839, "SPARC4_AC in"=w10840) -> ("error out"=w10847:errorcluster, "Sync Box.lvclass"=w10848:refnum<class "Sync Box.lvclass">, "SPARC4_AC out"=w10844:refnum<class "S4GUI.lvclass">)  [unwired: 7 in]
        n4579 = call-dynamic "Read Trigger.lvclass.vi"("error in (no error)"=w10847, "Sync Box in"=w10848) -> ("error out"=w10836:errorcluster, "Trigger.lvclass"=w10837:refnum<class "Trigger.lvclass">, "Sync Box out"=w10846:refnum<class "Sync Box.lvclass">)  [unwired: 7 in]
        n4580 = call-dynamic "Write DelayA.vi"("error in (no error)"=w10836, "DelayA"=w10835, "Trigger in"=w10837) -> ("error out"=w10842:errorcluster, "Trigger out"=w10841:refnum<class "Trigger.lvclass">)  [unwired: 7 in]
        n4581 = call-dynamic "Write Trigger.lvclass.vi"("error in (no error)"=w10842, "Trigger.lvclass"=w10841, "Sync Box in"=w10846) -> ("error out"=w10843:errorcluster, "Sync Box out"=w10845:refnum<class "Sync Box.lvclass">)  [unwired: 7 in]
        n4582 = call-dynamic "Write Sync Box.lvclass.vi"("error in (no error)"=w10843, "Sync Box.lvclass"=w10845, "SPARC4_AC in"=w10844) -> ("error out"=w10838:errorcluster, "SPARC4_AC out"=w10834:refnum<class "S4GUI.lvclass">)  [unwired: 7 in]
      }
      event "DelayB": Value Change {
        n4583 = event-data() -> ("NewVal"=w10850:string)  [unwired: 1 in, 3 out]
        n4584 = call-dynamic "Read Sync Box.lvclass.vi"("error in (no error)"=w10854, "SPARC4_AC in"=w10855) -> ("error out"=w10862:errorcluster, "Sync Box.lvclass"=w10863:refnum<class "Sync Box.lvclass">, "SPARC4_AC out"=w10859:refnum<class "S4GUI.lvclass">)  [unwired: 7 in]
        n4585 = call-dynamic "Read Trigger.lvclass.vi"("error in (no error)"=w10862, "Sync Box in"=w10863) -> ("error out"=w10851:errorcluster, "Trigger.lvclass"=w10852:refnum<class "Trigger.lvclass">, "Sync Box out"=w10861:refnum<class "Sync Box.lvclass">)  [unwired: 7 in]
        n4586 = call-dynamic "Write DelayB.vi"("error in (no error)"=w10851, "DelayB"=w10850, "Trigger in"=w10852) -> ("error out"=w10857:errorcluster, "Trigger out"=w10856:refnum<class "Trigger.lvclass">)  [unwired: 7 in]
        n4587 = call-dynamic "Write Trigger.lvclass.vi"("error in (no error)"=w10857, "Trigger.lvclass"=w10856, "Sync Box in"=w10861) -> ("error out"=w10858:errorcluster, "Sync Box out"=w10860:refnum<class "Sync Box.lvclass">)  [unwired: 7 in]
        n4588 = call-dynamic "Write Sync Box.lvclass.vi"("error in (no error)"=w10858, "Sync Box.lvclass"=w10860, "SPARC4_AC in"=w10859) -> ("error out"=w10853:errorcluster, "SPARC4_AC out"=w10849:refnum<class "S4GUI.lvclass">)  [unwired: 7 in]
      }
      event "DelayC": Value Change {
        n4589 = event-data() -> ("NewVal"=w10865:string)  [unwired: 1 in, 3 out]
        n4590 = call-dynamic "Read Sync Box.lvclass.vi"("error in (no error)"=w10869, "SPARC4_AC in"=w10870) -> ("error out"=w10877:errorcluster, "Sync Box.lvclass"=w10878:refnum<class "Sync Box.lvclass">, "SPARC4_AC out"=w10874:refnum<class "S4GUI.lvclass">)  [unwired: 7 in]
        n4591 = call-dynamic "Read Trigger.lvclass.vi"("error in (no error)"=w10877, "Sync Box in"=w10878) -> ("error out"=w10866:errorcluster, "Trigger.lvclass"=w10867:refnum<class "Trigger.lvclass">, "Sync Box out"=w10876:refnum<class "Sync Box.lvclass">)  [unwired: 7 in]
        n4592 = call-dynamic "Write DelayC.vi"("error in (no error)"=w10866, "DelayC"=w10865, "Trigger in"=w10867) -> ("error out"=w10872:errorcluster, "Trigger out"=w10871:refnum<class "Trigger.lvclass">)  [unwired: 7 in]
        n4593 = call-dynamic "Write Trigger.lvclass.vi"("error in (no error)"=w10872, "Trigger.lvclass"=w10871, "Sync Box in"=w10876) -> ("error out"=w10873:errorcluster, "Sync Box out"=w10875:refnum<class "Sync Box.lvclass">)  [unwired: 7 in]
        n4594 = call-dynamic "Write Sync Box.lvclass.vi"("error in (no error)"=w10873, "Sync Box.lvclass"=w10875, "SPARC4_AC in"=w10874) -> ("error out"=w10868:errorcluster, "SPARC4_AC out"=w10864:refnum<class "S4GUI.lvclass">)  [unwired: 7 in]
      }
      event "DelayD": Value Change {
        n4595 = event-data() -> ("NewVal"=w10880:string)  [unwired: 1 in, 3 out]
        n4596 = call-dynamic "Read Sync Box.lvclass.vi"("error in (no error)"=w10884, "SPARC4_AC in"=w10885) -> ("error out"=w10892:errorcluster, "Sync Box.lvclass"=w10893:refnum<class "Sync Box.lvclass">, "SPARC4_AC out"=w10889:refnum<class "S4GUI.lvclass">)  [unwired: 7 in]
        n4597 = call-dynamic "Read Trigger.lvclass.vi"("error in (no error)"=w10892, "Sync Box in"=w10893) -> ("error out"=w10881:errorcluster, "Trigger.lvclass"=w10882:refnum<class "Trigger.lvclass">, "Sync Box out"=w10891:refnum<class "Sync Box.lvclass">)  [unwired: 7 in]
        n4598 = call-dynamic "Write DelayD.vi"("error in (no error)"=w10881, "DelayD"=w10880, "Trigger in"=w10882) -> ("error out"=w10887:errorcluster, "Trigger out"=w10886:refnum<class "Trigger.lvclass">)  [unwired: 7 in]
        n4599 = call-dynamic "Write Trigger.lvclass.vi"("error in (no error)"=w10887, "Trigger.lvclass"=w10886, "Sync Box in"=w10891) -> ("error out"=w10888:errorcluster, "Sync Box out"=w10890:refnum<class "Sync Box.lvclass">)  [unwired: 7 in]
        n4600 = call-dynamic "Write Sync Box.lvclass.vi"("error in (no error)"=w10888, "Sync Box.lvclass"=w10890, "SPARC4_AC in"=w10889) -> ("error out"=w10883:errorcluster, "SPARC4_AC out"=w10879:refnum<class "S4GUI.lvclass">)  [unwired: 7 in]
      }
      event "WidthA": Value Change {
        n4601 = event-data() -> ("NewVal"=w10895:string)  [unwired: 1 in, 3 out]
        n4602 = call-dynamic "Read Sync Box.lvclass.vi"("error in (no error)"=w10899, "SPARC4_AC in"=w10900) -> ("error out"=w10907:errorcluster, "Sync Box.lvclass"=w10908:refnum<class "Sync Box.lvclass">, "SPARC4_AC out"=w10904:refnum<class "S4GUI.lvclass">)  [unwired: 7 in]
        n4603 = call-dynamic "Read Trigger.lvclass.vi"("error in (no error)"=w10907, "Sync Box in"=w10908) -> ("error out"=w10896:errorcluster, "Trigger.lvclass"=w10897:refnum<class "Trigger.lvclass">, "Sync Box out"=w10906:refnum<class "Sync Box.lvclass">)  [unwired: 7 in]
        n4604 = call-dynamic "Write WidthA.vi"("error in (no error)"=w10896, "WidthA"=w10895, "Trigger in"=w10897) -> ("error out"=w10902:errorcluster, "Trigger out"=w10901:refnum<class "Trigger.lvclass">)  [unwired: 7 in]
        n4605 = call-dynamic "Write Trigger.lvclass.vi"("error in (no error)"=w10902, "Trigger.lvclass"=w10901, "Sync Box in"=w10906) -> ("error out"=w10903:errorcluster, "Sync Box out"=w10905:refnum<class "Sync Box.lvclass">)  [unwired: 7 in]
        n4606 = call-dynamic "Write Sync Box.lvclass.vi"("error in (no error)"=w10903, "Sync Box.lvclass"=w10905, "SPARC4_AC in"=w10904) -> ("error out"=w10898:errorcluster, "SPARC4_AC out"=w10894:refnum<class "S4GUI.lvclass">)  [unwired: 7 in]
      }
      event "WidthB": Value Change {
        n4607 = event-data() -> ("NewVal"=w10910:string)  [unwired: 1 in, 3 out]
        n4608 = call-dynamic "Read Sync Box.lvclass.vi"("error in (no error)"=w10914, "SPARC4_AC in"=w10915) -> ("error out"=w10922:errorcluster, "Sync Box.lvclass"=w10923:refnum<class "Sync Box.lvclass">, "SPARC4_AC out"=w10919:refnum<class "S4GUI.lvclass">)  [unwired: 7 in]
        n4609 = call-dynamic "Read Trigger.lvclass.vi"("error in (no error)"=w10922, "Sync Box in"=w10923) -> ("error out"=w10911:errorcluster, "Trigger.lvclass"=w10912:refnum<class "Trigger.lvclass">, "Sync Box out"=w10921:refnum<class "Sync Box.lvclass">)  [unwired: 7 in]
        n4610 = call-dynamic "Write WidthB.vi"("error in (no error)"=w10911, "WidthB"=w10910, "Trigger in"=w10912) -> ("error out"=w10917:errorcluster, "Trigger out"=w10916:refnum<class "Trigger.lvclass">)  [unwired: 7 in]
        n4611 = call-dynamic "Write Trigger.lvclass.vi"("error in (no error)"=w10917, "Trigger.lvclass"=w10916, "Sync Box in"=w10921) -> ("error out"=w10918:errorcluster, "Sync Box out"=w10920:refnum<class "Sync Box.lvclass">)  [unwired: 7 in]
        n4612 = call-dynamic "Write Sync Box.lvclass.vi"("error in (no error)"=w10918, "Sync Box.lvclass"=w10920, "SPARC4_AC in"=w10919) -> ("error out"=w10913:errorcluster, "SPARC4_AC out"=w10909:refnum<class "S4GUI.lvclass">)  [unwired: 7 in]
      }
      event "WidthC": Value Change {
        n4613 = event-data() -> ("NewVal"=w10925:string)  [unwired: 1 in, 3 out]
        n4614 = call-dynamic "Read Sync Box.lvclass.vi"("error in (no error)"=w10929, "SPARC4_AC in"=w10930) -> ("error out"=w10937:errorcluster, "Sync Box.lvclass"=w10938:refnum<class "Sync Box.lvclass">, "SPARC4_AC out"=w10934:refnum<class "S4GUI.lvclass">)  [unwired: 7 in]
        n4615 = call-dynamic "Read Trigger.lvclass.vi"("error in (no error)"=w10937, "Sync Box in"=w10938) -> ("error out"=w10926:errorcluster, "Trigger.lvclass"=w10927:refnum<class "Trigger.lvclass">, "Sync Box out"=w10936:refnum<class "Sync Box.lvclass">)  [unwired: 7 in]
        n4616 = call-dynamic "Write WidthC.vi"("error in (no error)"=w10926, "WidthC"=w10925, "Trigger in"=w10927) -> ("error out"=w10932:errorcluster, "Trigger out"=w10931:refnum<class "Trigger.lvclass">)  [unwired: 7 in]
        n4617 = call-dynamic "Write Trigger.lvclass.vi"("error in (no error)"=w10932, "Trigger.lvclass"=w10931, "Sync Box in"=w10936) -> ("error out"=w10933:errorcluster, "Sync Box out"=w10935:refnum<class "Sync Box.lvclass">)  [unwired: 7 in]
        n4618 = call-dynamic "Write Sync Box.lvclass.vi"("error in (no error)"=w10933, "Sync Box.lvclass"=w10935, "SPARC4_AC in"=w10934) -> ("error out"=w10928:errorcluster, "SPARC4_AC out"=w10924:refnum<class "S4GUI.lvclass">)  [unwired: 7 in]
      }
      event "WidthD": Value Change {
        n4619 = event-data() -> ("NewVal"=w10940:string)  [unwired: 1 in, 3 out]
        n4620 = call-dynamic "Read Sync Box.lvclass.vi"("error in (no error)"=w10944, "SPARC4_AC in"=w10945) -> ("error out"=w10952:errorcluster, "Sync Box.lvclass"=w10953:refnum<class "Sync Box.lvclass">, "SPARC4_AC out"=w10949:refnum<class "S4GUI.lvclass">)  [unwired: 7 in]
        n4621 = call-dynamic "Read Trigger.lvclass.vi"("error in (no error)"=w10952, "Sync Box in"=w10953) -> ("error out"=w10941:errorcluster, "Trigger.lvclass"=w10942:refnum<class "Trigger.lvclass">, "Sync Box out"=w10951:refnum<class "Sync Box.lvclass">)  [unwired: 7 in]
        n4622 = call-dynamic "Write WidthD.vi"("error in (no error)"=w10941, "WidthD"=w10940, "Trigger in"=w10942) -> ("error out"=w10947:errorcluster, "Trigger out"=w10946:refnum<class "Trigger.lvclass">)  [unwired: 7 in]
        n4623 = call-dynamic "Write Trigger.lvclass.vi"("error in (no error)"=w10947, "Trigger.lvclass"=w10946, "Sync Box in"=w10951) -> ("error out"=w10948:errorcluster, "Sync Box out"=w10950:refnum<class "Sync Box.lvclass">)  [unwired: 7 in]
        n4624 = call-dynamic "Write Sync Box.lvclass.vi"("error in (no error)"=w10948, "Sync Box.lvclass"=w10950, "SPARC4_AC in"=w10949) -> ("error out"=w10943:errorcluster, "SPARC4_AC out"=w10939:refnum<class "S4GUI.lvclass">)  [unwired: 7 in]
      }
      event "WPROT_set": Value Change {
        # "Espera até 10 x 1s = 10s\npara condition de WPROT\n ir para READY"
        n4625 = event-data() -> ()  [unwired: 1 in, 4 out]
        n4626 = call "Read Instrument.lvclass.vi"("error in (no error)"=w10975, "S4ACS_GUI in"=w10976) -> ("error out"=w10973:errorcluster, "Instrument.lvclass"=w10974:refnum<class "Instrument.lvclass">, "S4ACS_GUI out"=w10962:refnum<class "S4GUI.lvclass">)  [unwired: 7 in]
